vi "Get XY Plot.vi"(8 "error in (no error)":errorcluster, 10 "Channel":u8, 11 "Micron sm Digitizer in":refnum<class "Micron sm Digitizer.lvclass">) -> (0 "error out":errorcluster, 2 "XY Plot":T1(graph), 3 "Micron sm Digitizer out":refnum<class "Micron sm Digitizer.lvclass">)   [LabVIEW 2024, in "Micron sm Digitizer.lvclass"]
uses:
  Micron sm Digitizer.lvclass
  Micron sm Digitizer.lvclass/Micron sm Digitizer.ctl
  Read VISA resource name.vi
  Write VISA resource name.vi
  Strain/Micron Optics sm130/Micron Optics sm130.lvlib
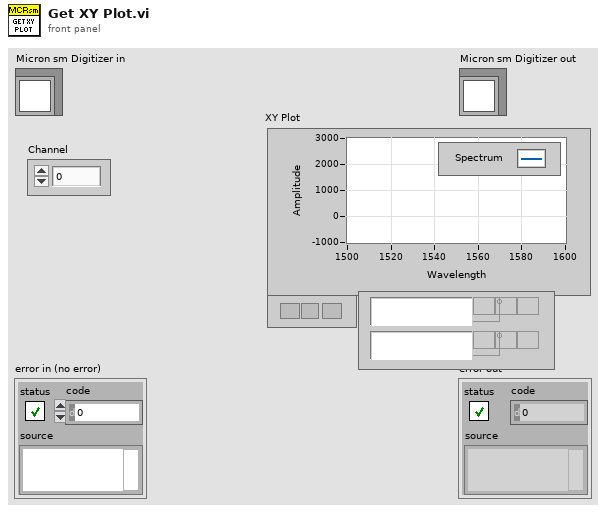
[diagram p1: front panel]
types:
  T1 = cluster{"Wavelength (nm)":dbl[], "Spectrum":dbl[]}[]
  T2 = cluster{"Wavelength (nm)":dbl[], "Spectrum":i16[]}[]
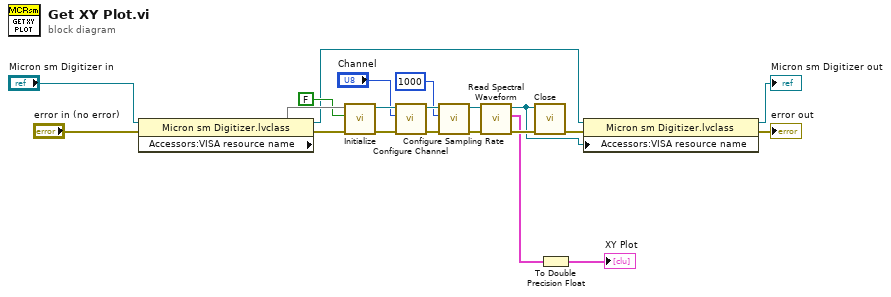
[diagram p0: block diagram]
diagram:
  n1 = property class="Micron sm Digitizer.lvclass"(reference="Micron sm Digitizer in", error in="error in (no error)") -> (reference out=w6:refnum<class "Micron sm Digitizer.lvclass">, error out=w14:errorcluster, "Accessors:VISA resource name"=w15)
  n2 = call "Initialize.vi"("error in (no error)"=w14, "ID Query (True)"=FALSE, "VISA resource name"=w15) -> ("error out"=w17:errorcluster, "VISA resource name out"=w16:refnum<visa-resource-name>)  [unwired: 7 in]
  n3 = call "Configure Channel.vi"("error in (no error)"=w17, "Channel (1: Channel 1)"="Channel", "VISA resource name"=w16) -> ("error out"=w19:errorcluster, "VISA resource name out"=w18:refnum<visa-resource-name>)  [unwired: 7 in]
  n4 = call "Configure Sampling Rate.vi"("error in (no error)"=w19, "Sample Rate (1000 Hz)"=1000, "VISA resource name"=w18) -> ("error out"=w10:errorcluster, "VISA resource name out"=w11:refnum<visa-resource-name>)  [unwired: 7 in]
  n5 = call "Read Spectral Waveform.vi"("error in (no error)"=w10, "VISA resource name"=w11) -> ("error out"=w9:errorcluster, "Spectral Waveform"=w2:T2, "VISA resource name out"=w7:refnum<visa-resource-name>)  [unwired: 7 in]
  n6 = call "Close.vi"("error in (no error)"=w9, "VISA resource name"=w7) -> ("error out"=w4:errorcluster)  [unwired: 9 in]
  n7 = To Double Precision Float(number=w2) -> (double precision float=→"XY Plot":T1)
  n8 = property class="Micron sm Digitizer.lvclass"(reference=w6, error in=w4, "Accessors:VISA resource name"=w7) -> (reference out=→"Micron sm Digitizer out":refnum<class "Micron sm Digitizer.lvclass">, error out=→"error out":errorcluster)
